vi "Stop DC_X_Brake.vi"   [LabVIEW 2010, in "4134Outputs.lvlib"]
uses:
  4134Outputs.lvlib
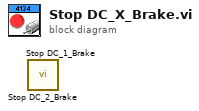
[diagram p0: block diagram]
diagram:
  n1 = call "Stop DC_2_Brake.vi"() -> ()  [unwired: 10 in, 1 out]
  n2 = call "Stop DC_1_Brake.vi"() -> ()  [unwired: 10 in, 1 out]
